vi "MoveX.vi"(8 "error in (no error)":errorcluster, 10 "Left?":bool, 11 "PongPanel in":refnum<class "PongPanel.lvclass">) -> (0 "error out":errorcluster, 3 "PongPanel out":refnum<class "PongPanel.lvclass">)   [LabVIEW 2019, in "RT_Game.lvlib" / "PongPanel.lvclass"]
uses:
  PongPanel.lvclass
  C:/Users/FreshBob/Dropbox/VIs/myRIO_GameConsole/RT/RT_Game/GameObject/GameObject.lvclass
  GameObject/GameObject.lvclass/GameObject.ctl
  PongPanel.lvclass/PongPanel.ctl
  GameObject/Read position.vi
  GameObject/Read size.vi
  GameObject/Write position.vi
  Globals.vi
  RT_Game.lvlib
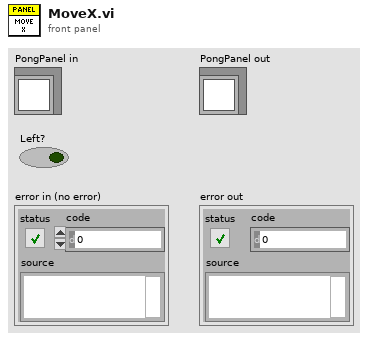
[diagram p1: front panel]
types:
  T1 = typedef "RT_Game.lvlib/Game.lvclass/Coordinate.ctl" = cluster{"x":dbl, "y":dbl}
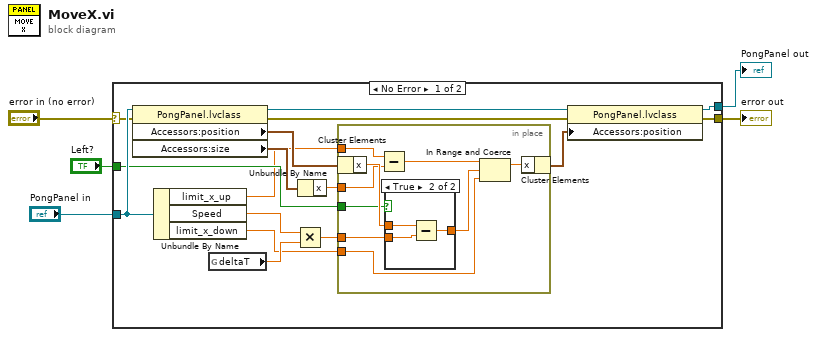
[diagram p0: block diagram]
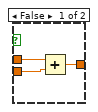
[diagram p2: hidden frame]
diagram:
  n1 = case shown="No Error" "error in (no error)" {
    selector: "error in (no error)" -> [w15 w38]
    tunnel: [w14 w38] -> w2
    tunnel: [w17 w37] -> w4
    tunnel: "PongPanel in" -> [w21 w37]
    tunnel: "Left?" -> [w8 _]
    frame No Error {
      n2 = property class="PongPanel.lvclass"(reference=w21, error in=w15) -> (reference out=w18:refnum<class "PongPanel.lvclass">, error out=w16:errorcluster, "Accessors:position"=w13:T1, "Accessors:size"=w10:T1)
      n3 = Unbundle By Name(w21) -> ("limit_x_up"=w7:dbl, "Speed"=w20:dbl, "limit_x_down"=w6:dbl)
      n4 = global read "Globals.vi" "deltaT"() -> (w19:dbl)
      n5 = Multiply(x=w20, y=w19) -> (x*y=w11:dbl)
      n6 = Unbundle By Name(w10) -> ("x"=w9:dbl)
      n7 = in-place {
        in-place-border: w11 -> [w29]
        in-place-border: w7 -> [w25]
        in-place-border: w9 -> [w24]
        in-place-border: w8 -> [w27]
        in-place-border: w6 -> [w22]
        n8 = in-place-cluster #1(w13) -> ("x"=w30:dbl)
        n9 = Subtract(x=w25, y=w24) -> (x-y=w23:dbl)
        n10 = case shown="True" w27 {
          tunnel: w30 -> [w33 w36]
          tunnel: w29 -> [w32 w35]
          tunnel: [w31 w34] -> w28
          frame False {
            n11 = Add(x=w33, y=w32) -> (x+y=w31:dbl)
          }
          frame True {
            n12 = Subtract(x=w36, y=w35) -> (x-y=w34:dbl)
          }
        }
        n13 = In Range and Coerce(upper limit=w23, x=w28, lower limit=w22) -> (coerced(x)=w26:dbl)  [unwired: 1 out]
        n14 = in-place-cluster #1("x"=w26) -> (w12:T1)
      }
      n15 = property class="PongPanel.lvclass"(reference=w18, error in=w16, "Accessors:position"=w12) -> (reference out=w17:refnum<class "PongPanel.lvclass">, error out=w14:errorcluster)
    }
    frame Error {
    }
  }
  "PongPanel out" <- w4
  "error out" <- w2
